vi "rs3 start self-cal.vi"(7 "error in (no error)":errorcluster, 9 "Speed (0-3, 1 default)":i32, 10 "device in":u64) -> (0 "error out":errorcluster, 1 "error":u64, 3 "Device out":u64, 4 "result (0=success)":i32)   [LabVIEW 2017, in "libRealSense3.lvlib"]
doc: "Starts the on-chip self-calibration process. \nUse the Get Self-Cal Status to see results, and the Burn_Self_cal to burn this to flash so it persists. \n\nparam[in] device RealSense device\nparam[in] speed 0 Very fast, 1 Fast, 2 Medium, 3 Slow\nparam[out] error if non-null, receives any error that occurs during this call, otherwise, errors are ignored\n\nreturn true if succeeded"
uses:
  libRealSense3.lvlib
  realsense2.dll
panel:
  # "RS3 Start Self-Cal"
  # "(C) Intel Corp. 2019,  AGJ"
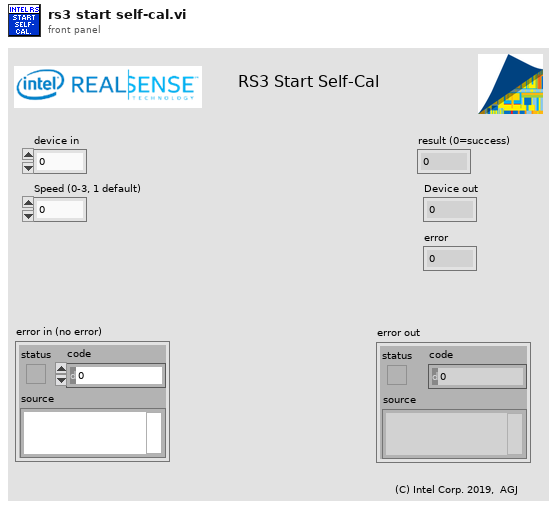
[diagram p1: front panel]
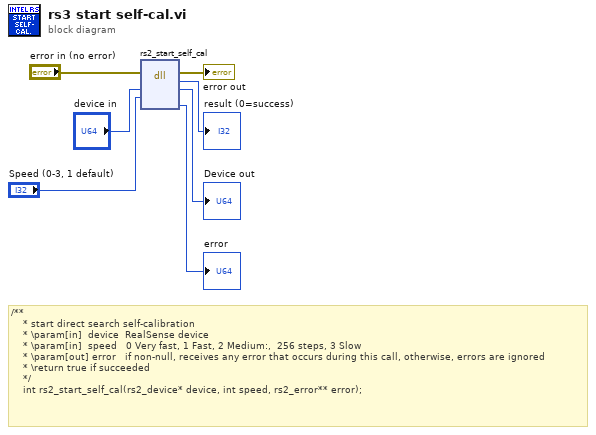
[diagram p0: block diagram]
diagram:
  # "/**\n    * start direct search self-calibration\n    * \\param[in]  device  RealSense device\n    * \\param[in]  speed   0 Very fast, 1 Fast, 2 Medium:,  256 steps, 3 Slow\n    * \\param[out] error   if non-null, receives any error that occurs during this call, otherwise, errors are ignored\n    * \\return true if succeeded\n    */\n    int rs2_start_self_cal(rs2_device* device, int speed, rs2_error** error);"
  n1 = dll-call lib="C:/Users/agrunnet/Documents/libRealSense6/realsense2.dll" fn="rs2_start_self_cal"(error in="error in (no error)", "device"="device in", "speed"="Speed (0-3, 1 default)") -> (error out=→"error out":errorcluster, "result"=→"result (0=success)":i32, "device"=→"Device out":u64, "error"=→"error":u64)  [unwired: 4 in, 1 out]
